vi "LoginBaru.vi"(8 "error in (no error)":errorcluster, 11 "connection information":path=path "D:/TUBES_SCADA_FIX/database.udl") -> (0 "error out 2":errorcluster, 1 "Role":string, 3 "Cancel":bool)   [LabVIEW 2025]
uses:
  <vilib>/Alab Technologies/AES Crypto/Public VIs/String to Array.vi
  <vilib>/Alab Technologies/AES Crypto/Public VIs/Array to String.vi
  <vilib>/addons/database/Connection.llb/DB Tools Open Connec (Path).vi
  <vilib>/addons/database/NI_Database_API.lvlib
  <vilib>/Alab Technologies/AES Crypto/AES Crypto.lvlib
panel:
  out "Data sama?":bool
  out "RePassword Hex":string
  out "Password Hax":string
  out "error out 4":errorcluster
  out "Role DB":string
  out "Username DB":string
  in  "error in (no error) 2":errorcluster
  out "Data 0?":bool
  out "error out 3":errorcluster
  out "Hasil Query 2":string
  out "Password":string
  out "Username":string
  out "OK Button 2":bool
  in  "Stop Button":bool
  in  "Multicolumn Listbox":i32(listbox)
  out "error out":errorcluster
  out "Hasil Query":string
  in  "Tab Control":enum32{"Page 1", "Page 3", "Page 2"}(tab)
  in  "Lupa psw":bool
  in  "Close Button":bool
  in  "OK Button":bool
  in  "Password":string
  in  "Username":string
  in  "Set Password":bool
  in  "Password Baru":string
  in  "Role":string
  in  "Username":string
  in  "Close Button 2":bool
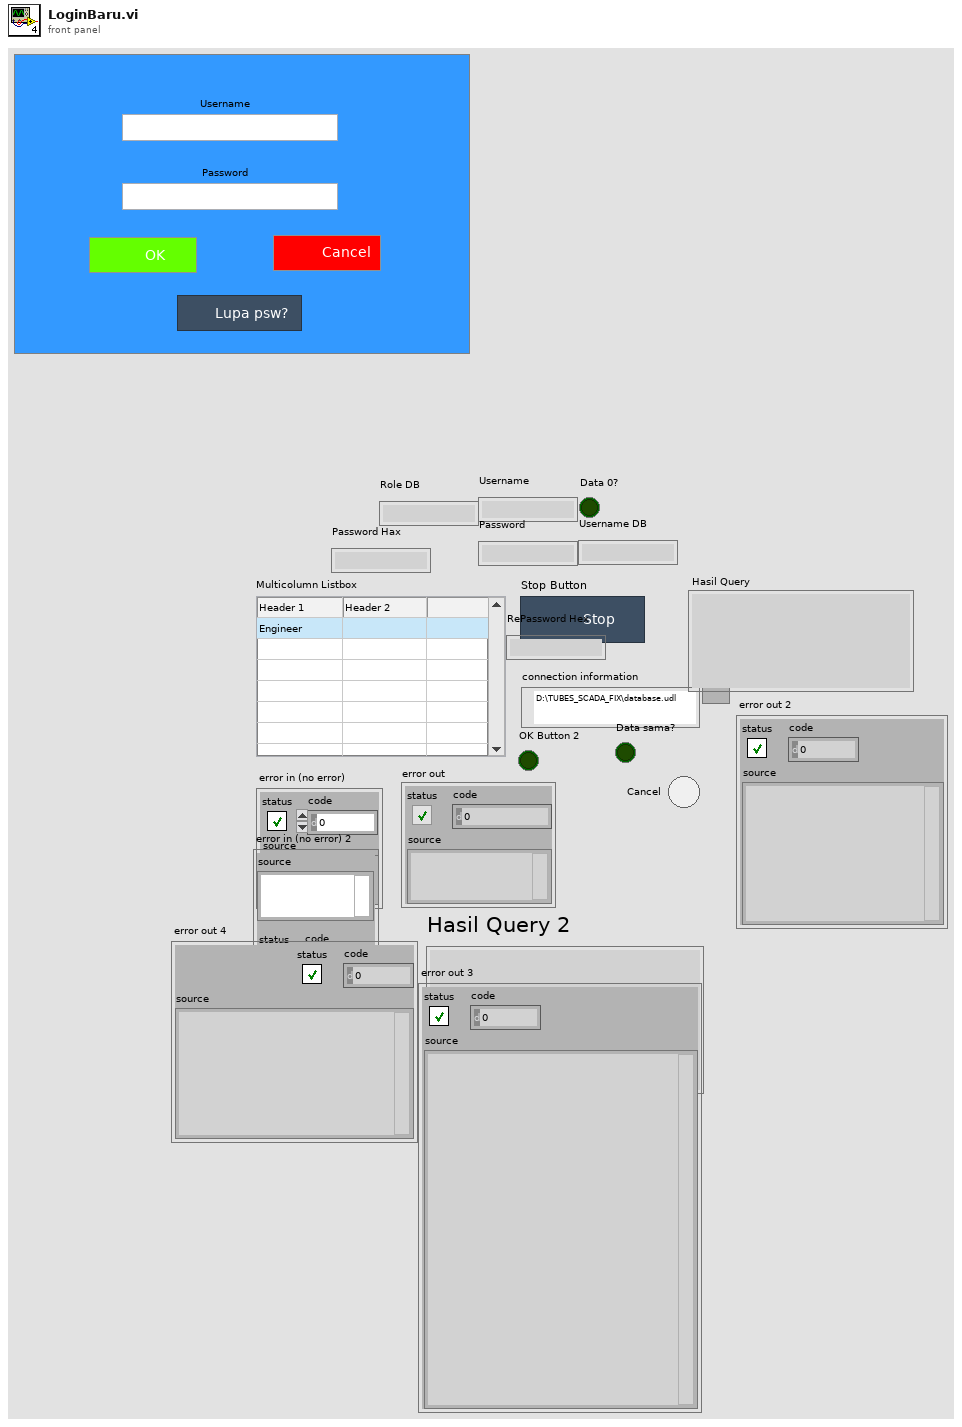
[diagram p1: front panel]
types:
  T1 = typedef "NI_Database_API.lvlib/Conn ObjectReference.ctl" = refnum<k1>
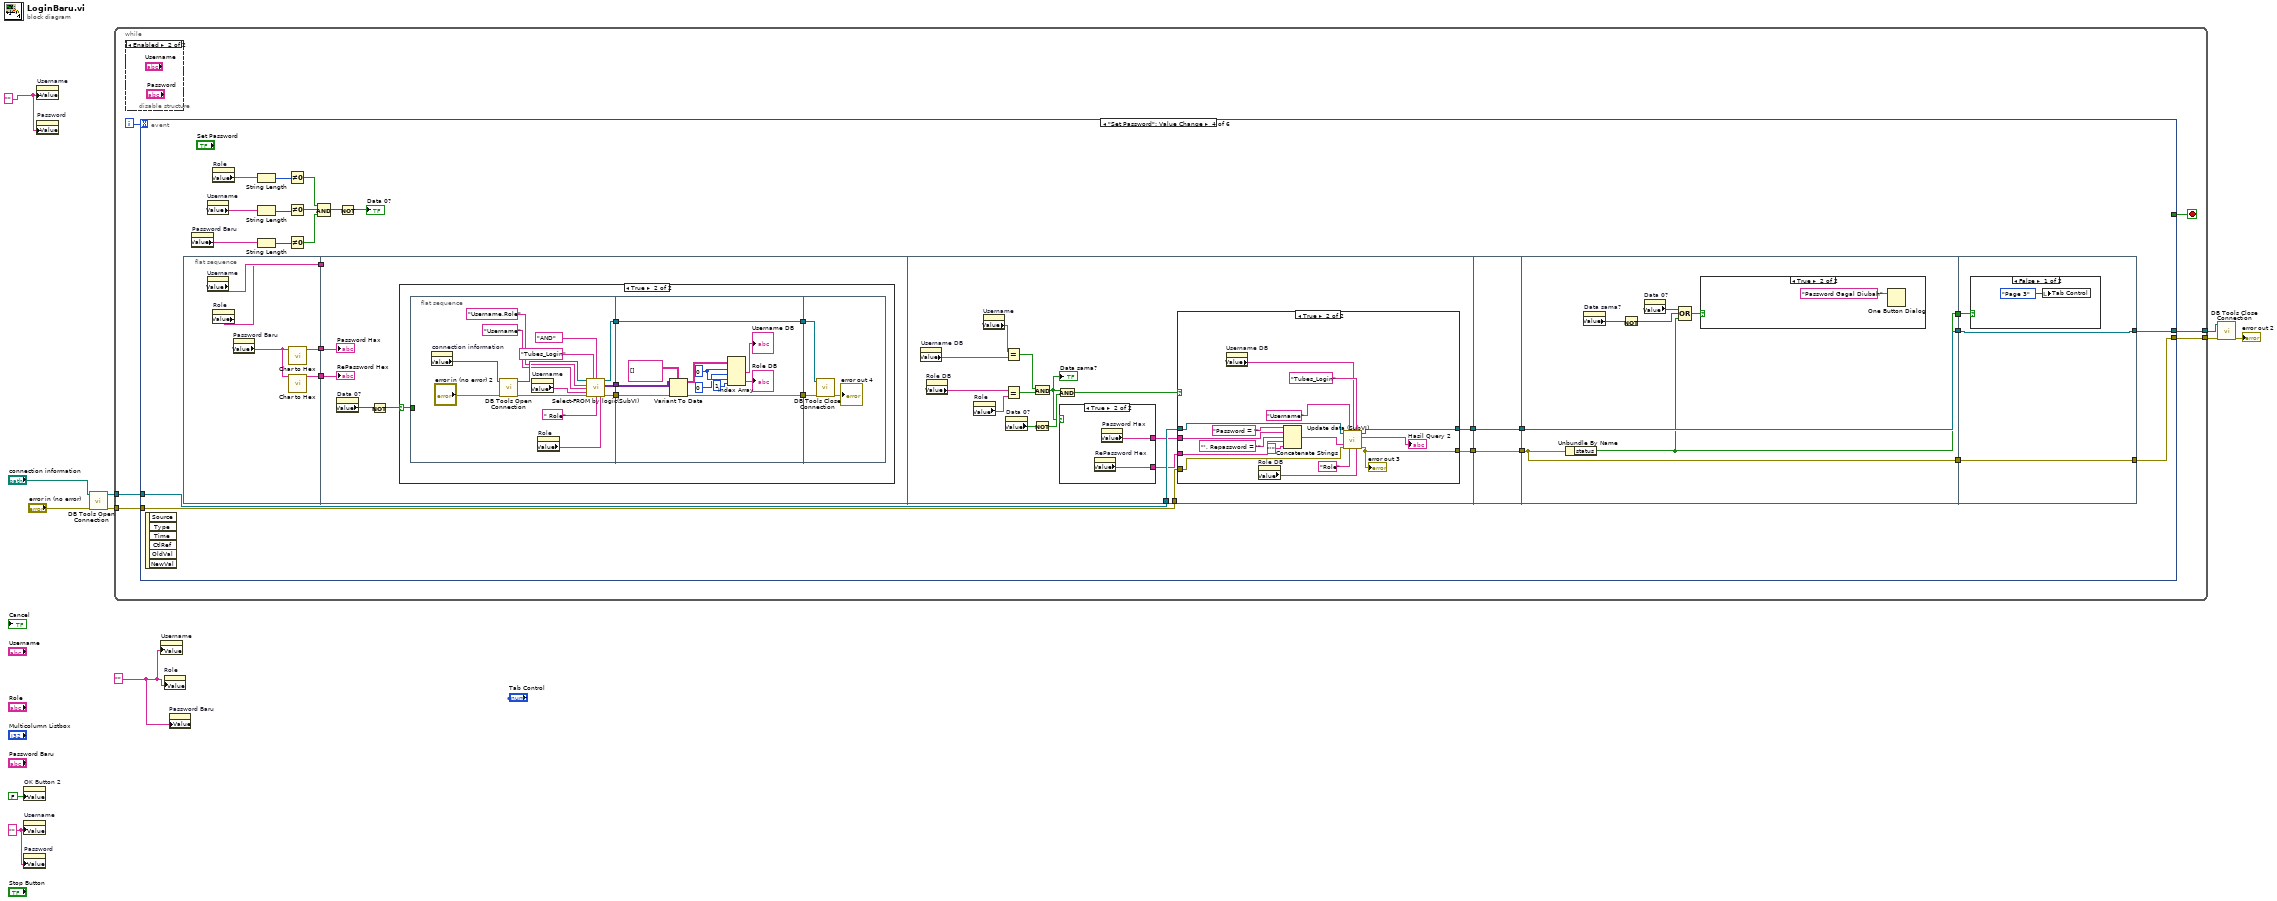
[diagram p0: block diagram]
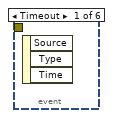
[diagram p3: hidden frame]
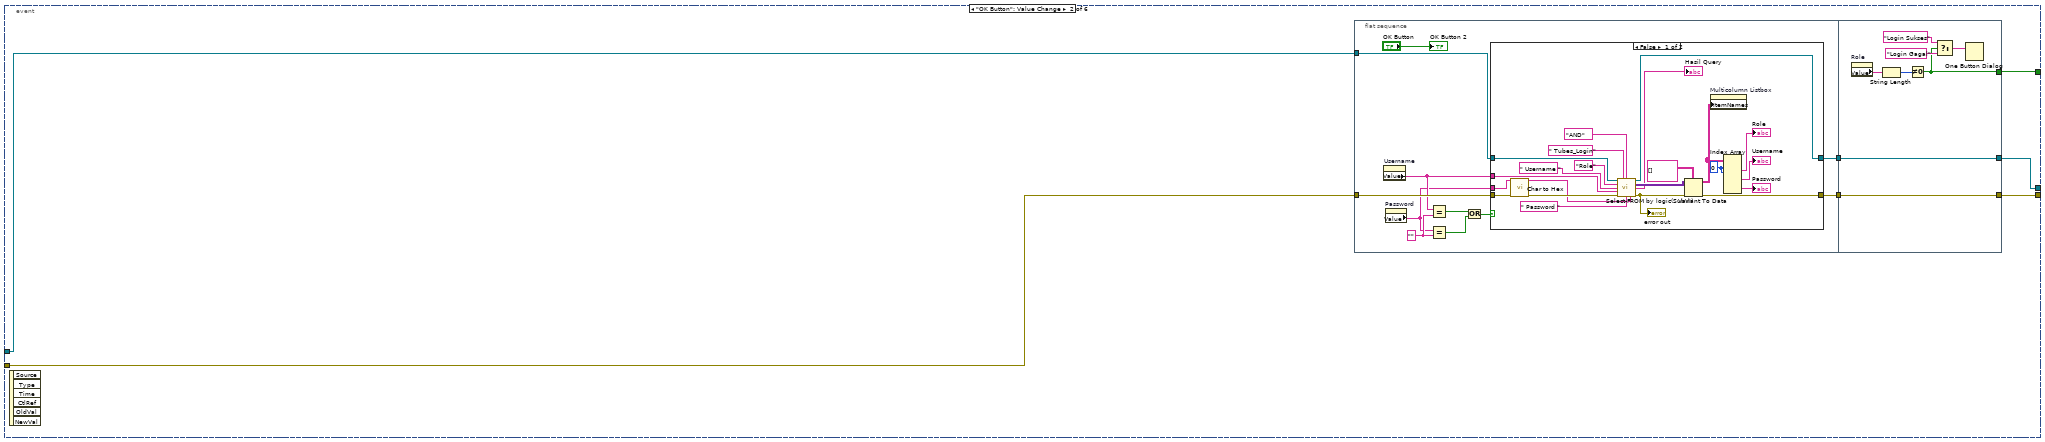
[diagram p4: hidden frame]
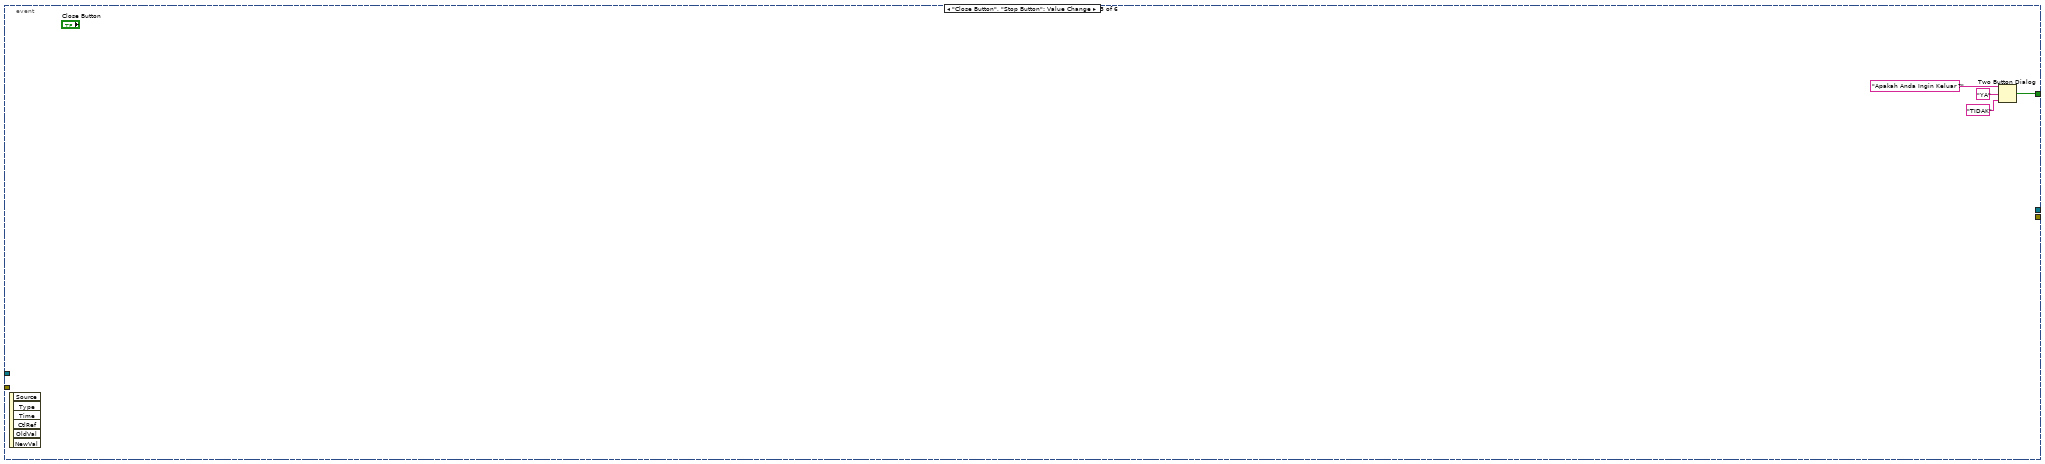
[diagram p6: hidden frame]
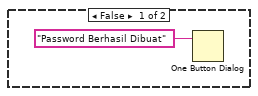
[diagram p10: hidden frame]
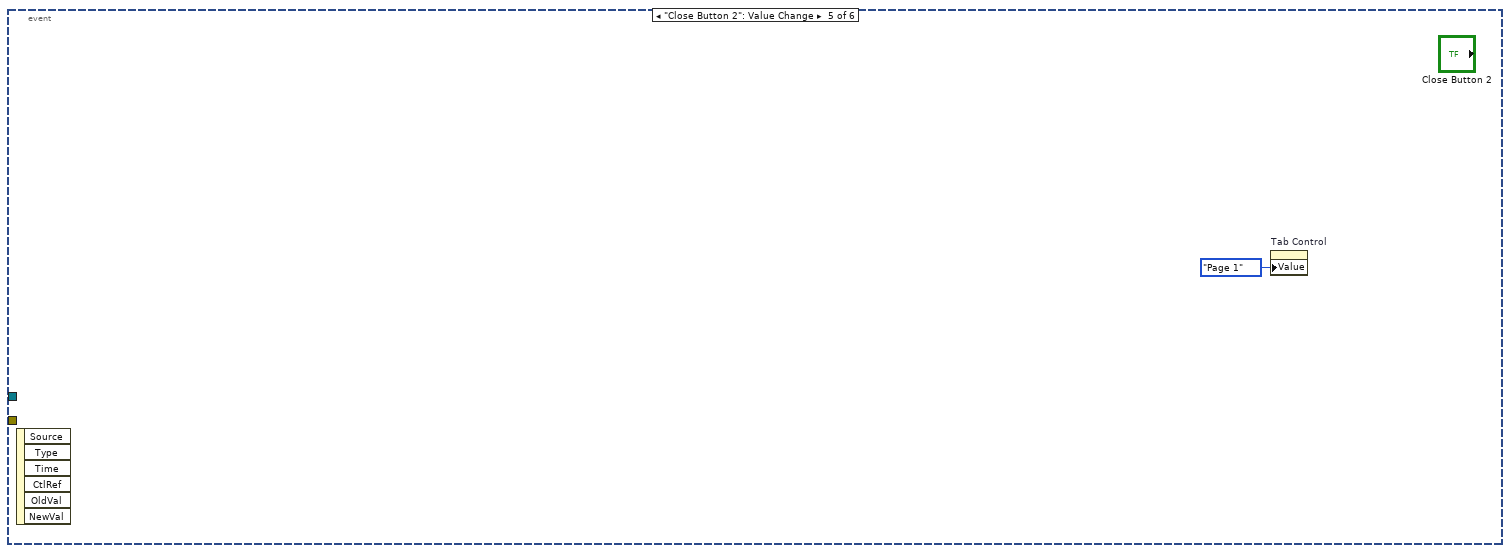
[diagram p12: hidden frame]
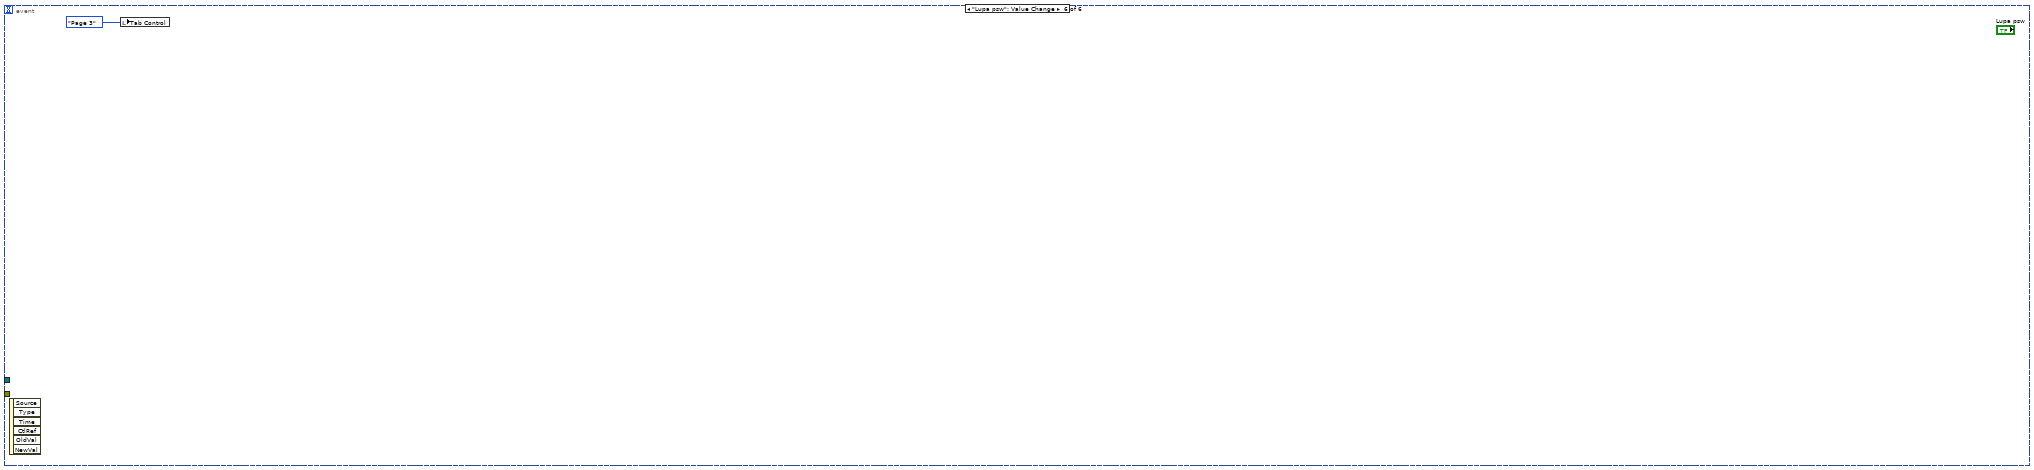
[diagram p13: hidden frame]
diagram:
  w1 = ""
  w2 = ""
  w6 = ""
  n1 = property on="OK Button 2" class="Bool (strict)"("Value"=FALSE ("OK Button 2")) -> ()  [unwired: 2 in, 2 out]
  n2 = property on="Username" class="Str"("Value"=w6) -> ()  [unwired: 2 in, 2 out]
  n3 = property on="Password" class="Str"("Value"=w6) -> ()  [unwired: 2 in, 2 out]
  n4 = property on="Username" class="Str"("Value"=w1) -> ()  [unwired: 2 in, 2 out]
  n5 = property on="Password" class="Str"("Value"=w1) -> ()  [unwired: 2 in, 2 out]
  n6 = call-poly <vilib>:"DB Tools Open Connection.vi"("error in (no error)"="error in (no error)", "connection information"="connection information") -> ("error out"=w9:errorcluster, "connection reference"=w8:T1)  [unwired: 6 in]
  n7 = while {
    tunnel: w9 -> [w15]
    tunnel: w8 -> [w14]
    tunnel: [w13] -> w4
    tunnel: [w12] -> w3
    i -> [w17]
    stop <- w16 stop-if-true
    n8 = disable-structure shown="Enabled" {
      frame Disabled {
      }
      frame Enabled {
      }
    }
    n9 = event shown="[3] \"Set Password\": Value Change" {
      selector: _ -> [_ _ _ _ _ _]
      dyn-events: _ -> [_ _ _ _ _ _]
      timeout: w17 -> [_ _ _ _ _ _]
      tunnel: [_ w22 w68 _ _ _] -> w16
      tunnel: w15 -> [_ w24 _ w97 _ _]
      tunnel: w14 -> [_ w23 _ w96 _ _]
      tunnel: [_ w20 _ w92 _ _] -> w13
      tunnel: [_ w18 _ w91 _ _] -> w12
      event Timeout {
        n10 = event-data() -> ()  [unwired: 1 in, 3 out]
      }
      event "OK Button": Value Change {
        n11 = event-data() -> ()  [unwired: 1 in, 6 out]
        n12 = flat-sequence {
          tunnel: w24 -> [w30]
          tunnel: w23 -> [w31]
          tunnel: [w29] -> w21
          tunnel: [w28] -> w19
          tunnel: [w63] -> w22
          tunnel: w21 -> [w60]
          tunnel: [w61] -> w20
          tunnel: w19 -> [w61]
          tunnel: [w60] -> w18
          frame #0 {
            w32 = ""
            n13 = property on="Username" class="Str"() -> ("Value"=w26:string)  [unwired: 2 in, 2 out]
            n14 = property on="Password" class="Str"() -> ("Value"=w25:string)  [unwired: 2 in, 2 out]
            n15 = Equal?(x=w26, y=w32) -> (x = y?=w34:bool)
            n16 = Equal?(x=w25, y=w32) -> (x = y?=w33:bool)
            n17 = Or(x=w34, y=w33) -> (x .or. y?=w27:bool)
            n18 = case shown="False" w27 {
              tunnel: w31 -> [w45 w59]
              tunnel: w30 -> [w43 w58]
              tunnel: [w44 w59] -> w29
              tunnel: [w36 w58] -> w28
              tunnel: w26 -> [w41 _]
              tunnel: w25 -> [w40 _]
              frame False {
                w47 = 0
                n19 = call <vilib>:"Char to Hex.vi"("Input string (char)"=w40, "error in (no error)"=w43) -> ("Output string (hex)"=w39:string, "error out"=w42:errorcluster)  [unwired: 12 in]
                n20 = call "Select-FROM by logic(SubVI).vi"("connection reference"=w45, "TABLE"=" Tubes_Login", "Logic data"="AND", "COLOUM 1"="Role", "COLOUM Data 1"=" Username " ("Nilai 1"), "Nilai 1"=w41, "error in (no error)"=w42, "COLOUM Data 2"=" Password ", "Nilai 2"=w39) -> ("connection reference 2"=w44:T1, "recordset data"=w55:variant[][], "Hasil Query"=→"Hasil Query":string, "error out"=w54:errorcluster)  [unwired: 2 in, 1 out]
                "error out" <- w54
                n21 = Variant To Data(error in=w54, type=string[][] [], Variant=w55) -> (data=w57:string[][], error out=w36:errorcluster)
                n22 = property on="Multicolumn Listbox" class="MCListbox (strict)"("ItemNames"=w57) -> ()  [unwired: 2 in, 2 out]
                n23 = Index Array(array=w57, index (row) #1=w47, index (col) #1=w47) -> (element #1=→"Role":string, element #2=→"Username":string, element #3=→"Password":string)  [unwired: 4 in]
              }
              frame True {
              }
            }
            "OK Button 2" <- "OK Button"
          }
          frame #1 {
            n24 = property on="Role" class="Str"() -> ("Value"=w67:string)  [unwired: 2 in, 2 out]
            n25 = String Length(string=w67) -> (length=w66:i32)
            n26 = Not Equal To 0?(x=w66) -> (x != 0?=w63:bool)
            n27 = Select(t="Login Sukses", s=w63, f="Login Gagal") -> (s? t:f=w62:string)
            n28 = One Button Dialog(message=w62) -> ()  [unwired: 1 in, 1 out]
          }
        }
      }
      event "Close Button", "Stop Button": Value Change {
        n29 = event-data() -> ()  [unwired: 1 in, 6 out]
        n30 = Two Button Dialog(message="Apakah Anda Ingin Keluar ?", 1:"TIDAK" ("F button name (\"Cancel\")"), 2:"YA" ("T button name (\"OK\")")) -> (T button?=w68:bool)
      }
      event "Set Password": Value Change {
        n31 = event-data() -> ()  [unwired: 1 in, 6 out]
        n32 = flat-sequence {
          tunnel: [w101] -> w75
          tunnel: [w100] -> w74
          tunnel: [w99] -> w73
          tunnel: [w98] -> w72
          tunnel: w75 -> [w104]
          tunnel: w74 -> [w103]
          tunnel: w73 -> [_]
          tunnel: w72 -> [_]
          tunnel: w97 -> [w156]
          tunnel: w96 -> [w155]
          tunnel: [w154] -> w90
          tunnel: [w153] -> w88
          tunnel: w90 -> [w178]
          tunnel: [w178] -> w89
          tunnel: w88 -> [w177]
          tunnel: [w177] -> w80
          tunnel: w89 -> [w185]
          tunnel: [w182] -> w95
          tunnel: [w185] -> w94
          tunnel: [w184] -> w93
          tunnel: w80 -> [w184]
          tunnel: w95 -> [w190]
          tunnel: [w189] -> w92
          tunnel: w94 -> [w189]
          tunnel: [w188] -> w91
          tunnel: w93 -> [w188]
          frame #0 {
            n33 = property on="Username" class="Str"() -> ("Value"=w99:string)  [unwired: 2 in, 2 out]
            n34 = property on="Role" class="Str"() -> ("Value"=w98:string)  [unwired: 2 in, 2 out]
            n35 = property on="Password Baru" class="Str"() -> ("Value"=w102:string)  [unwired: 2 in, 2 out]
            n36 = call <vilib>:"Char to Hex.vi"("Input string (char)"=w102) -> ("Output string (hex)"=w101:string)  [unwired: 13 in, 1 out]
            n37 = call <vilib>:"Char to Hex.vi"("Input string (char)"=w102) -> ("Output string (hex)"=w100:string)  [unwired: 13 in, 1 out]
          }
          frame #1 {
            n38 = property on="Data 0?" class="Bool (strict)"() -> ("Value"=w106:bool)  [unwired: 2 in, 2 out]
            n39 = Not(x=w106) -> (.not. x?=w105:bool)
            n40 = case shown="True" w105 {
              selector: w105 -> [_ w112]
              frame False {
              }
              frame True {
                n41 = flat-sequence {
                  tunnel: w112 -> [_]
                  tunnel: [w117] -> w111
                  tunnel: [w116] -> w110
                  tunnel: [w115] -> w109
                  tunnel: w111 -> [w132]
                  tunnel: w110 -> [w133]
                  tunnel: w109 -> [w128]
                  tunnel: [w128] -> w108
                  tunnel: [w127] -> w107
                  tunnel: w108 -> [w140]
                  tunnel: w107 -> [w139]
                  frame #0 {
                    n42 = property on="connection information" class="Path"() -> ("Value"=w124:path)  [unwired: 2 in, 2 out]
                    n43 = call-poly <vilib>:"DB Tools Open Connection.vi"("error in (no error)"="error in (no error) 2", "connection information"=w124) -> ("error out"=w119:errorcluster, "connection reference"=w125:T1)  [unwired: 6 in]
                    n44 = property on="Username" class="Str"() -> ("Value"=w114:string)  [unwired: 2 in, 2 out]
                    n45 = property on="Role" class="Str"() -> ("Value"=w113:string)  [unwired: 2 in, 2 out]
                    n46 = call "Select-FROM by logic(SubVI).vi"("connection reference"=w125, "TABLE"="Tubes_Login" ("Nilai User"), "Logic data"="AND", "COLOUM 1"="Username,Role", "COLOUM Data 1"="Username", "Nilai 1"=w114, "error in (no error)"=w119, "COLOUM Data 2"=" Role", "Nilai 2"=w113) -> ("connection reference 2"=w115:T1, "recordset data"=w117:variant[][], "error out"=w116:errorcluster)  [unwired: 2 in, 2 out]
                  }
                  frame #1 {
                    w137 = 0 ("index (row)")
                    n47 = Variant To Data(error in=w133, type=string[][] [], Variant=w132) -> (data=w131:string[][], error out=w127:errorcluster)
                    n48 = Index Array(array=w131, index (row) #1=w137, index (col) #1=0 ("disabled index (col)"), index (row) #2=w137, index (col) #2=1 ("disabled index (col)")) -> (element #1=→"Username DB":string, element #2=→"Role DB":string)
                  }
                  frame #2 {
                    n49 = call <vilib>:"DB Tools Close Connection.vi"("error in (no error)"=w139, "connection reference"=w140) -> ("error out"=→"error out 4":errorcluster)  [unwired: 5 in]
                  }
                }
              }
            }
            "Password Hax" <- w104
            "RePassword Hex" <- w103
          }
          frame #2 {
            n50 = property on="Username DB" class="Str"() -> ("Value"=w150:string)  [unwired: 2 in, 2 out]
            n51 = property on="Role DB" class="Str"() -> ("Value"=w149:string)  [unwired: 2 in, 2 out]
            n52 = property on="Role" class="Str"() -> ("Value"=w148:string)  [unwired: 2 in, 2 out]
            n53 = property on="Username" class="Str"() -> ("Value"=w151:string)  [unwired: 2 in, 2 out]
            n54 = Equal?(x=w151, y=w150) -> (x = y?=w147:bool)
            n55 = Equal?(x=w149, y=w148) -> (x = y?=w146:bool)
            n56 = property on="Data 0?" class="Bool (strict)"() -> ("Value"=w152:bool)  [unwired: 2 in, 2 out]
            n57 = Not(x=w152) -> (.not. x?=w145:bool)
            n58 = And(x=w147, y=w146) -> (x .and. y?=w144:bool)
            "Data sama?" <- w144
            n59 = And(x=w144, y=w145) -> (x .and. y?=w143:bool)
            n60 = case shown="True" w144 {
              tunnel: [_ w158] -> w142
              tunnel: [_ w157] -> w141
              frame False {
              }
              frame True {
                n61 = property on="RePassword Hex" class="Str"() -> ("Value"=w157:string)  [unwired: 2 in, 2 out]
                n62 = property on="Password Hax" class="Str"() -> ("Value"=w158:string)  [unwired: 2 in, 2 out]
              }
            }
            n63 = case shown="True" w143 {
              tunnel: w156 -> [w159 w171]
              tunnel: w155 -> [w160 w170]
              tunnel: [w159 w168] -> w154
              tunnel: [w160 w167] -> w153
              tunnel: w142 -> [_ w166]
              tunnel: w141 -> [_ w165]
              frame False {
              }
              frame True {
                n64 = property on="Username DB" class="Str"() -> ("Value"=w162:string)  [unwired: 2 in, 2 out]
                n65 = property on="Role DB" class="Str"() -> ("Value"=w161:string)  [unwired: 2 in, 2 out]
                n66 = Concatenate Strings("Password = '" ("string"), w166, "', Repassword = '" ("string"), w165, "'" ("string")) -> (w163:string)
                n67 = call "Update data (SubVI).vi"("Refnum in"=w170, "Kolom Username"="Username", "Nilai User"=w162, "Nama Table"="Tubes_Login" ("Nilai User"), "Set Nilai"=w163, "error in (no error)"=w171, "Kolom Role"="Role", "Nilai Role"=w161) -> ("Refnum out"=w167:T1, "Hasil Query"=→"Hasil Query 2":string, "error out"=w168:errorcluster)  [unwired: 5 in]
                "error out 3" <- w168
              }
            }
          }
          frame #3 {
          }
          frame #4 {
            n68 = Unbundle By Name(w185) -> ("status"=w182:bool)
            n69 = property on="Data sama?" class="Bool (strict)"() -> ("Value"=w181:bool)  [unwired: 2 in, 2 out]
            n70 = Not(x=w181) -> (.not. x?=w180:bool)
            n71 = property on="Data 0?" class="Bool (strict)"() -> ("Value"=w183:bool)  [unwired: 2 in, 2 out]
            n72 = Compound Arithmetic op=OR(w183, w180, w182) -> (w179:bool)
            n73 = case shown="True" w179 {
              frame False {
                n74 = One Button Dialog(message="Password Berhasil Dibuat") -> ()  [unwired: 1 in, 1 out]
              }
              frame True {
                n75 = One Button Dialog(message="Password Gagal Diubah") -> ()  [unwired: 1 in, 1 out]
              }
            }
          }
          frame #5 {
            n76 = case shown="False" w190 {
              frame False {
                n77 = local write "Tab Control"(enum32{"Page 1", "Page 3", "Page 2"}."Page 3" ("Tab Control")) -> ()
              }
              frame True {
              }
            }
          }
        }
        n78 = property on="Password Baru" class="Str"() -> ("Value"=w84:string)  [unwired: 2 in, 2 out]
        n79 = property on="Username" class="Str"() -> ("Value"=w83:string)  [unwired: 2 in, 2 out]
        n80 = property on="Role" class="Str"() -> ("Value"=w82:string)  [unwired: 2 in, 2 out]
        n81 = String Length(string=w82) -> (length=w85:i32)
        n82 = String Length(string=w83) -> (length=w86:i32)
        n83 = String Length(string=w84) -> (length=w87:i32)
        n84 = Not Equal To 0?(x=w85) -> (x != 0?=w79:bool)
        n85 = Not Equal To 0?(x=w86) -> (x != 0?=w78:bool)
        n86 = Not Equal To 0?(x=w87) -> (x != 0?=w77:bool)
        n87 = Compound Arithmetic op=AND(w79, w78, w77) -> (w81:bool)
        n88 = Not(x=w81) -> (.not. x?=→"Data 0?":bool)
      }
      event "Close Button 2": Value Change {
        n89 = event-data() -> ()  [unwired: 1 in, 6 out]
        n90 = property on="Tab Control" class="TabCtl (strict)"("Value"=enum32{"Page 1", "Page 3", "Page 2"}."Page 1" ("Tab Control")) -> ()  [unwired: 2 in, 2 out]
      }
      event "Lupa psw": Value Change {
        n91 = event-data() -> ()  [unwired: 1 in, 6 out]
        n92 = local write "Tab Control"(enum32{"Page 1", "Page 3", "Page 2"}."Page 3" ("Tab Control")) -> ()
      }
    }
  }
  n93 = property on="Username" class="Str"("Value"=w2) -> ()  [unwired: 2 in, 2 out]
  n94 = property on="Role" class="Str"("Value"=w2) -> ()  [unwired: 2 in, 2 out]
  n95 = property on="Password Baru" class="Str"("Value"=w2) -> ()  [unwired: 2 in, 2 out]
  n96 = call <vilib>:"DB Tools Close Connection.vi"("error in (no error)"=w4, "connection reference"=w3) -> ("error out"=→"error out 2":errorcluster)  [unwired: 5 in]
